vi "verify operation mode.vi"(8 "error in (no error)":errorcluster, 11 "Channel in":refnum<class "SPARC4_Channel.lvclass">) -> (0 "error out":errorcluster, 3 "Channel out":refnum<class "SPARC4_Channel.lvclass">)   [LabVIEW 2018, in "SPARC4_Channel.lvclass"]
uses:
  SPARC4_Channel.lvclass
  Channel/Channel.lvclass
  Sim_Ixon_Ultra/Sim_Ixon_Ultra.lvclass
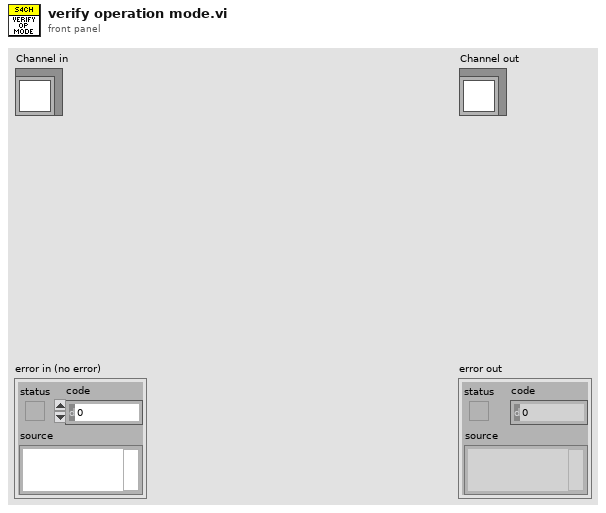
[diagram p1: front panel]
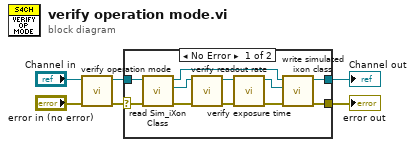
[diagram p0: block diagram]
diagram:
  n1 = call-parent "verify operation mode.vi"("error in (no error)"="error in (no error)", "Channel in"="Channel in") -> ("error out"=w2:errorcluster, "Channel out"=w3:refnum<class "SPARC4_Channel.lvclass">)  [unwired: 8 in]
  n2 = case shown="No Error" w2 {
    selector: w2 -> [w16 w19]
    tunnel: [w7 w19] -> w6
    tunnel: [w8 w18] -> w5
    tunnel: w3 -> [w17 w18]
    frame No Error {
      n3 = call "read Sim_iXon Class.vi"("error in (no error)"=w16, "SPARC4_Channel in"=w17) -> ("error out"=w15:errorcluster, "Sim_Ixon_Ultra.lvclass"=w13:refnum<class "Sim_Ixon_Ultra.lvclass">, "SPARC4_Channel out"=w14:refnum<class "SPARC4_Channel.lvclass">)  [unwired: 7 in]
      n4 = call "verify readout rate.vi"("error in (no error)"=w15, "Sim_Ixon_Ultra in"=w13) -> ("error out"=w12:errorcluster, "Sim_Ixon_Ultra out"=w9:refnum<class "Sim_Ixon_Ultra.lvclass">)  [unwired: 8 in]
      n5 = call-dynamic "verify exposure time.vi"("error in (no error)"=w12, "Simulated_CCD_Camera in"=w9) -> ("error out"=w11:errorcluster, "Simulated_CCD_Camera out"=w10:refnum<class "Sim_Ixon_Ultra.lvclass">)  [unwired: 8 in]
      n6 = call "write simulated ixon class.vi"("error in (no error)"=w11, "Sim_Ixon_Ultra.lvclass"=w10, "SPARC4_Channel in"=w14) -> ("error out"=w7:errorcluster, "SPARC4_Channel out"=w8:refnum<class "SPARC4_Channel.lvclass">)  [unwired: 7 in]
    }
    frame Error {
    }
  }
  "error out" <- w6
  "Channel out" <- w5
